vi "Main Board Game.vi"(8 "error in (no error)":errorcluster, 11 "Module_Refs":T1={"ModuleName"=enum."Controller", "Queue"=refnum, "user event"=refnum, "VI Refnum"=refnum, "ShowFP"=FALSE, "StatesTracking Enabled"=FALSE}) -> (0 "error out":errorcluster)   [LabVIEW 2021, in "Board Game.lvlib"]
doc: "Main Module Template of the architecture. Use this as a template to integrate new independent processes into your application."
uses:
  Board Game.lvlib
  Typedefs/Module References.ctl
  Typedefs/Enum_Module_Name.ctl
  Typedefs/Message.ctl
  Typedefs/State Machine Data.ctl
  Typedefs/Config.ctl
  Application/Game.lvclass
  Configuration/Typedefs/App Cfg DVR.ctl
  Typedefs/Application Configuration.ctl
  Module Template/Typedefs/Config.ctl
  Modules/Sound Manager/Typedefs/Config.ctl
  Core UI Configuraton Extractor API.vi
  Configuration/Configuration.lvlib
  Architecture.lvlib
  Module Template/Module Template.lvlib
  Modules/Sound Manager/Sound Manager.lvlib
panel:
  in  "Stop App":bool
  out "Message":string
  in  "Stop Module":bool
  # "#Architecture\n\nPlace inside this box all visible data."
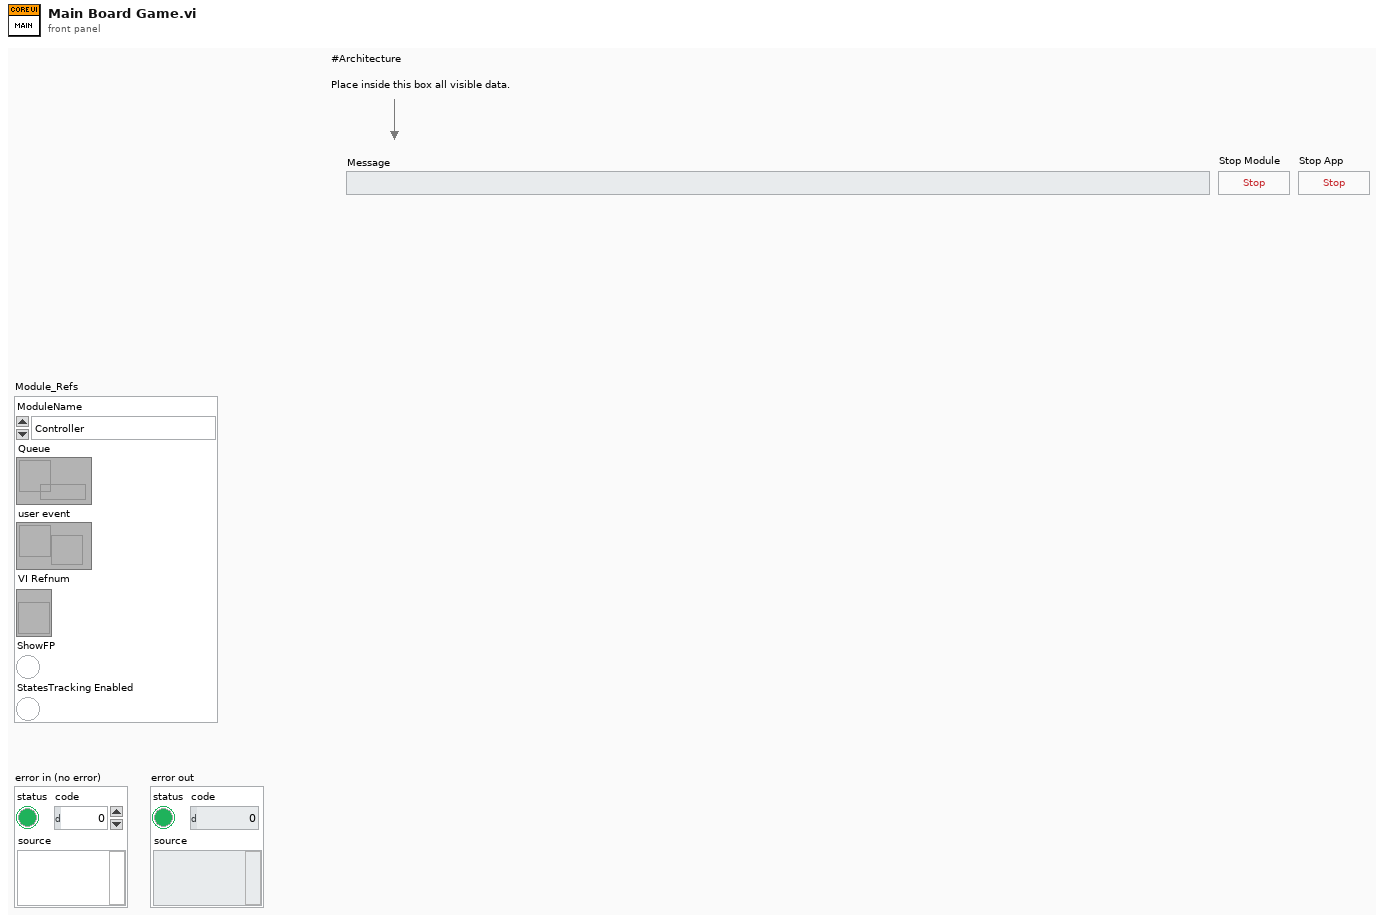
[diagram p1: front panel]
types:
  T1 = typedef "Architecture.lvlib/Module References.ctl" = cluster{"ModuleName":T2, "Queue":refnum<queue>, "user event":refnum<user-event>, "VI Refnum":refnum<vi>, "ShowFP":bool, "StatesTracking Enabled":bool}
  T2 = typedef "Configuration.lvlib/Enum_Module_Name.ctl" = enum16{"Configuration", "Error_Handler", "Log", "Database", "Controller", "UI Module", "Sound Manager"}
  T3 = typedef "Board Game.lvlib/State Machine Data.ctl" = cluster{"Module_Refs":T1, "Response Data":variant, "Core UI Config":T4, "Game":refnum<class "Game.lvclass">}
  T4 = typedef "Board Game.lvlib/Config.ctl" = cluster{"Module Enabled":bool}
  T5 = enum32{"Invalid", "Standard", "Closed", "Hidden", "Minimized", "Maximized"}
  T6 = typedef "Error_Manager.lvlib/LogRotate.lvclass/LogData.ctl" = cluster{"error in":errorcluster, "replacements":string[], "Time Stamp":timestamp}
  T7 = typedef "Configuration.lvlib/App Cfg DVR.ctl" = refnum<data-value>
  T8 = typedef "Module Template.lvlib/Config.ctl" = cluster{"Module Enabled":bool}
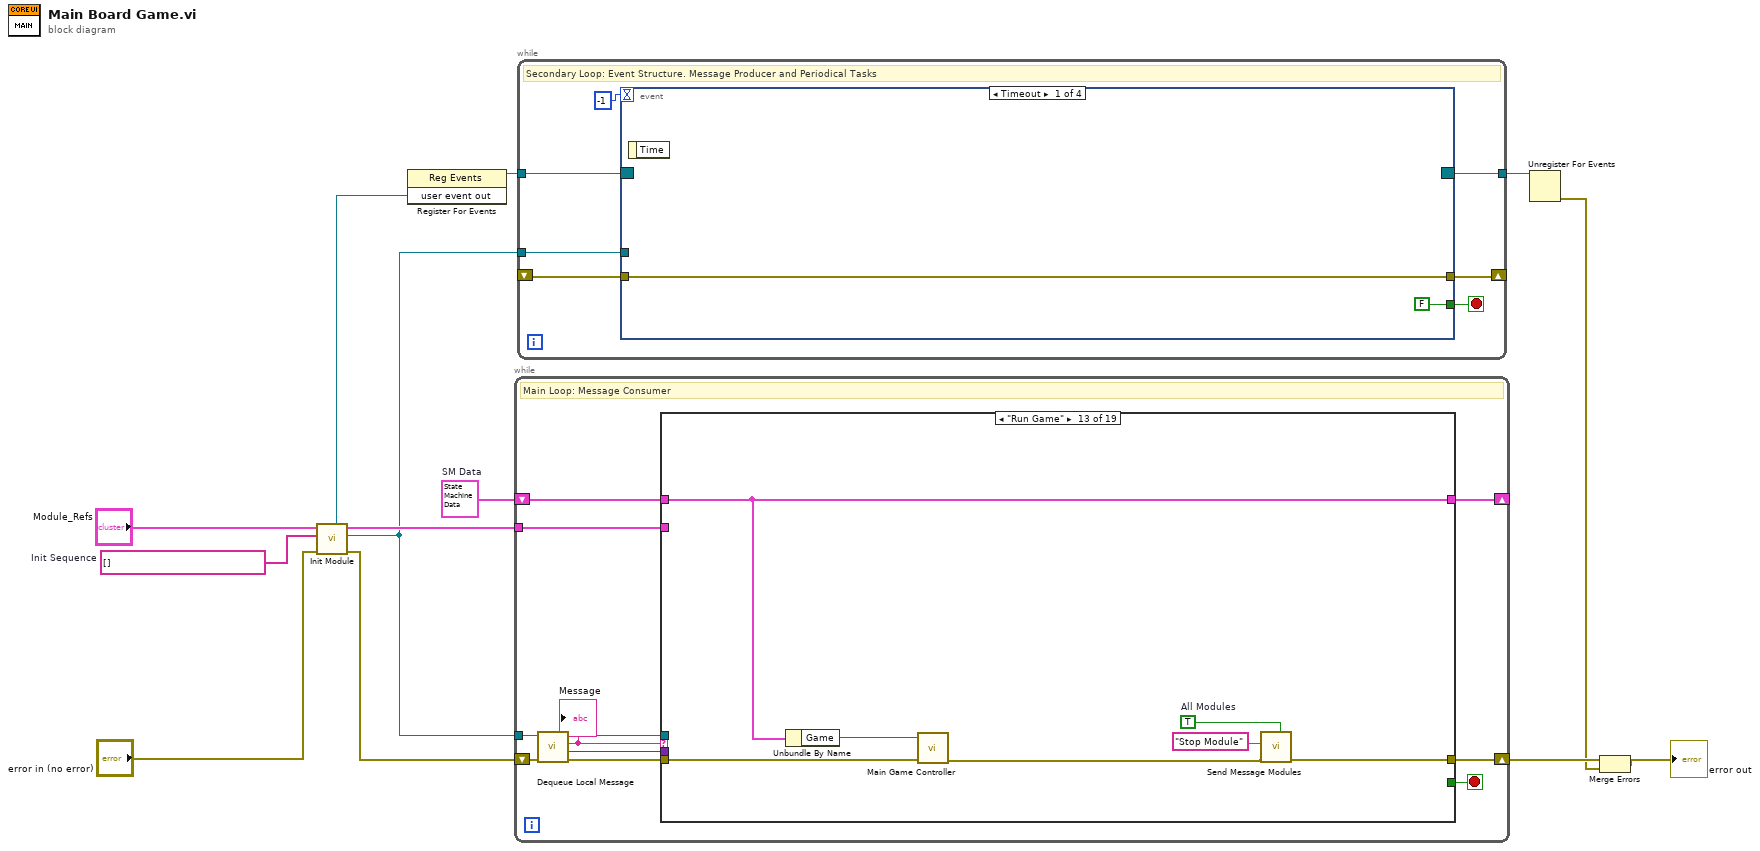
[diagram p0: block diagram]
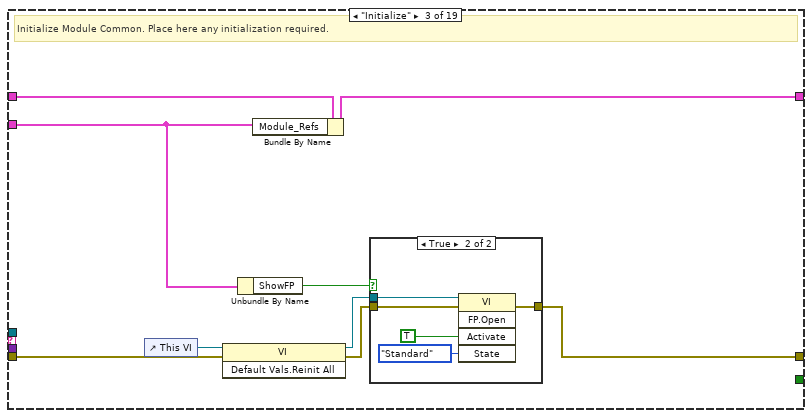
[diagram p4: hidden frame]
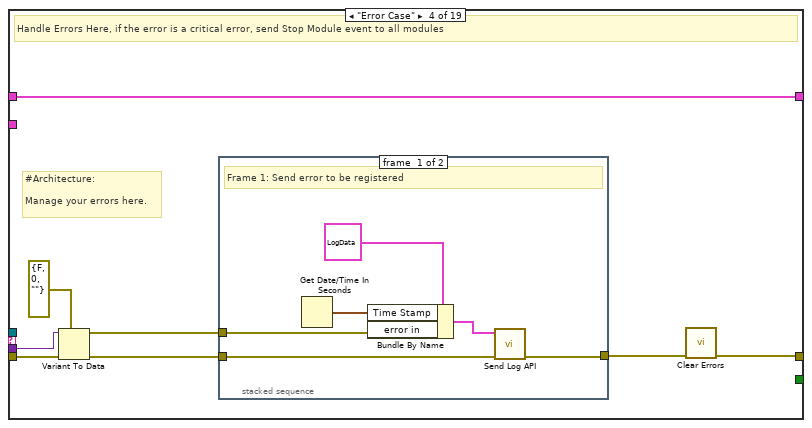
[diagram p6: hidden frame]
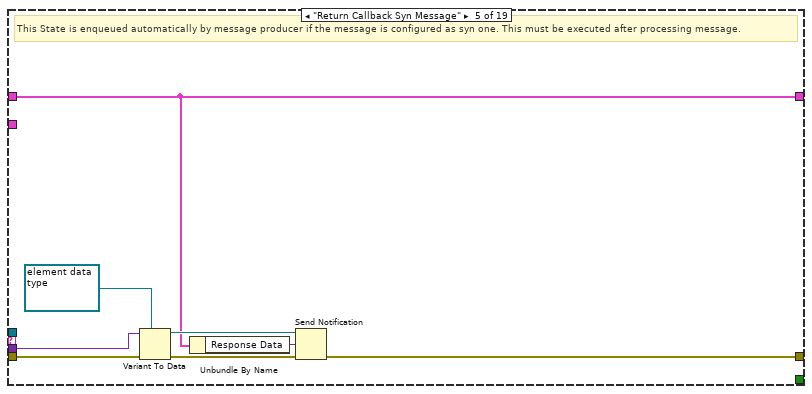
[diagram p9: hidden frame]
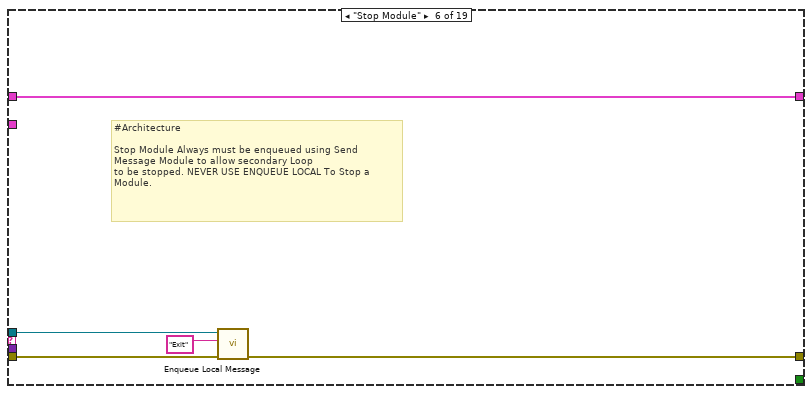
[diagram p10: hidden frame]
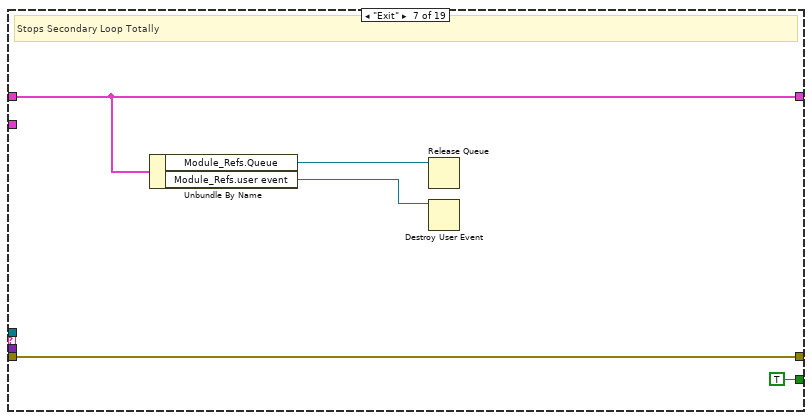
[diagram p11: hidden frame]
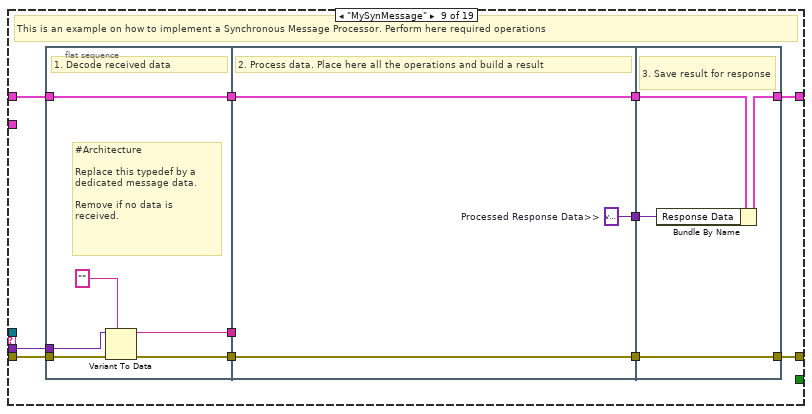
[diagram p13: hidden frame]
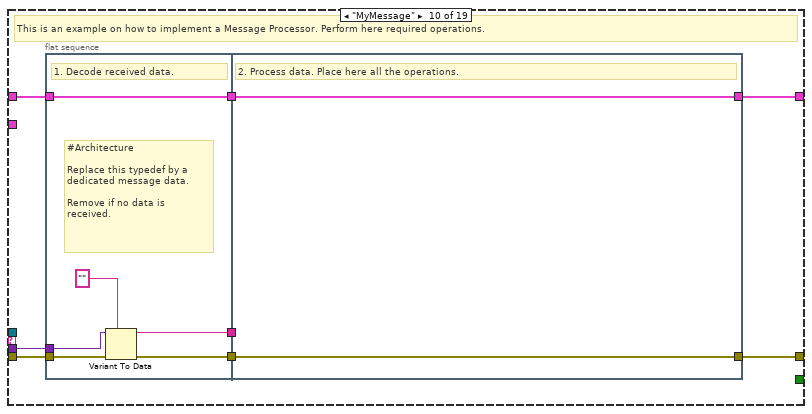
[diagram p14: hidden frame]
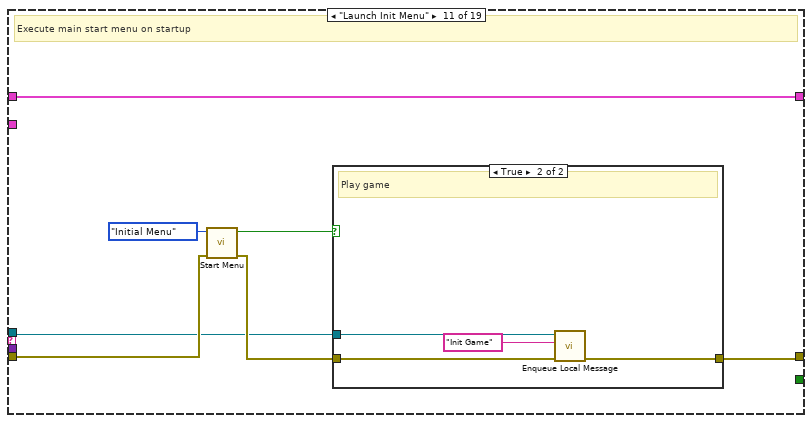
[diagram p15: hidden frame]
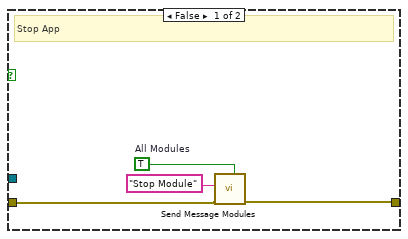
[diagram p16: hidden frame]
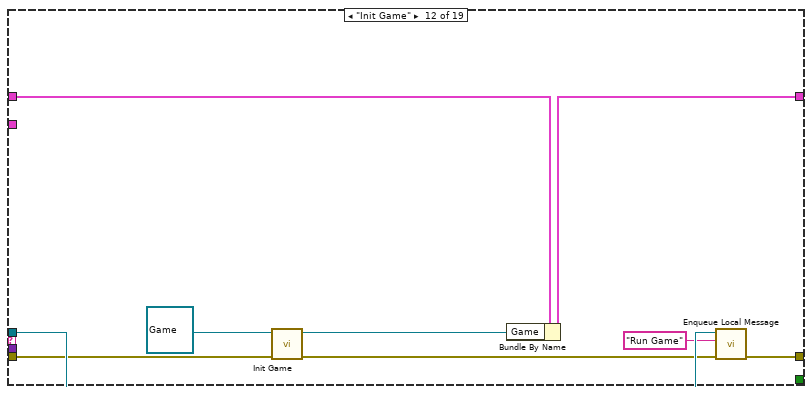
[diagram p17: hidden frame]
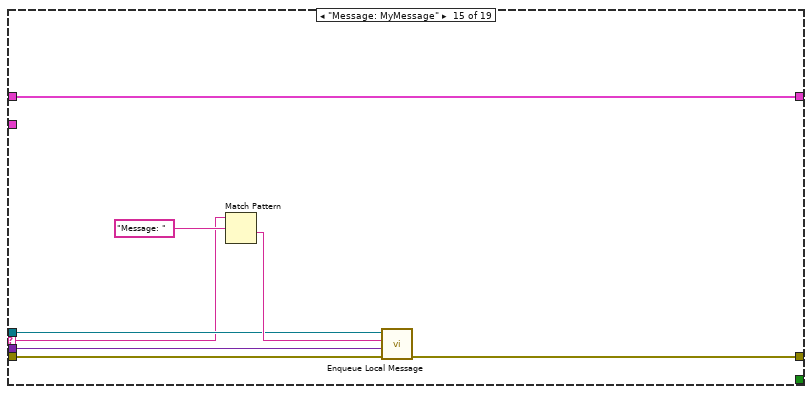
[diagram p19: hidden frame]
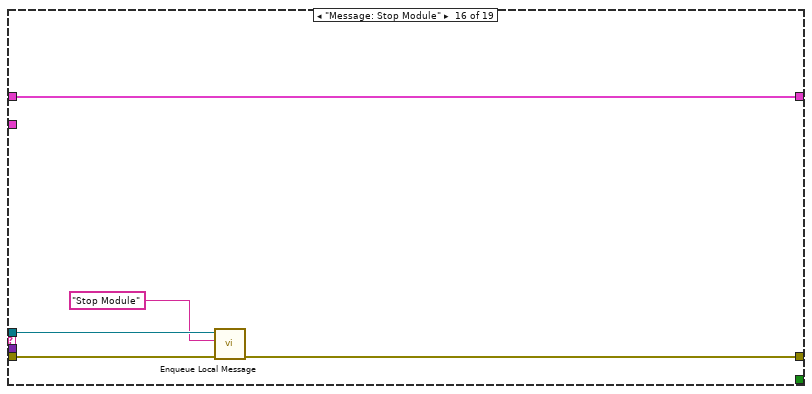
[diagram p20: hidden frame]
diagram:
  w10 = string[] []  # Init Sequence
  w13 = T3 {"Module_Refs"={"ModuleName"=enum."Configuration", "Queue"=refnum, "user event"=refnum, "VI Refnum"=refnum, "ShowFP"=FALSE, "StatesTracking Enabled"=FALSE}, "Response Data"=variant, "Core UI Config"={"Module Enabled"=FALSE}, "Game"=refnum}  # SM Data
  n1 = call "Init Module.vi"("error in (no error)"="error in (no error)", "Init Sequence"=w10, "Module Refs"="Module_Refs") -> ("error out"=w12:errorcluster, "queue out"=w1:refnum<queue>, "Module Refs Out"=w3:T1, "user event out"=w2:refnum<user-event>)  [unwired: 5 in]
  n2 = register-events(w2) -> (reference out=w9:refnum<event-registration>)  [unwired: 2 in, 1 out]
  n3 = while {
    shift-right: [w23] -> _
    shift-left: w13 -> [w24]
    shift-right: [w22] -> w7
    shift-left: w12 -> [w20]
    tunnel: w1 -> [w21]
    tunnel: w3 -> [w14]
    stop <- w15 stop-if-true
    # "Main Loop: Message Consumer"
    n4 = call "Dequeue Local Message.vi"("error in"=w20, "Msg queue in"=w21) -> ("error out"=w19:errorcluster, "Data"=w16:variant, "Message"=w17:string, "queue out"=w18:refnum<queue>)  [unwired: 6 in]
    "Message" <- w17
    n5 = case shown="\"Run Game\"" w17 {
      selector: w17 -> [_ _ _ _ _ _ _ _ _ _ _ _ _ _ w155 _ _ _ w187]
      tunnel: w24 -> [w26 w28 w37 w51 w63 w74 w77 w81 w92 w113 w128 w145 w152 w154 w162 w167 w176 w178 w192]
      tunnel: [w26 w28 w35 w51 w63 w74 w77 w81 w91 w106 w128 w144 w152 w154 w162 w167 w170 w178 w192] -> w23
      tunnel: w19 -> [w25 w27 w36 w50 w69 w73 w79 w80 w85 w109 w127 w138 w147 w153 w159 w166 w175 w177 w191]
      tunnel: [w25 w27 w31 w44 w68 w72 w79 w80 w90 w112 w123 w143 w146 w153 w156 w165 w171 w177 w181] -> w22
      tunnel: w18 -> [_ _ _ _ _ w71 _ _ _ _ w122 w142 _ _ w157 w164 _ _ w188]
      tunnel: w16 -> [_ _ _ w49 w66 _ _ _ w84 w108 _ _ _ _ w158 _ w174 _ w189]
      tunnel: [_ _ _ _ _ _ TRUE _ _ _ _ _ _ _ _ _ _ _ _] -> w15
      tunnel: w14 -> [_ _ w34 _ _ _ _ _ _ _ _ _ _ _ _ _ _ _ _]
      frame "--------State Machine Arquitechture Operations--------" {
      }
      frame "Idle", Default {
        # "Use this state to make iterations if required."
      }
      frame "Initialize" {
        # "Initialize Module Common. Place here any initialization required."
        n6 = control-ref of="This VI"() -> (w29:refnum<vi>)
        n7 = invoke class="VI" method="Default Vals.Reinit All"(reference=w29, error in=w36) -> (reference out=w32:refnum<vi>, error out=w33:errorcluster)  [unwired: 1 in, 1 out]
        n8 = Unbundle By Name(w34) -> ("ShowFP"=w30:bool)
        n9 = Bundle By Name(cluster=w37, "Module_Refs"=w34) -> (w35:T3)
        n10 = case shown="True" w30 {
          tunnel: w33 -> [w38 w43]
          tunnel: [w38 w42] -> w31
          tunnel: w32 -> [_ w41]
          frame False {
          }
          frame True {
            n11 = invoke class="VI" method="FP.Open"(reference=w41, error in=w43, "Activate"=TRUE ("Activate?"), "State"=T5."Standard") -> (error out=w42:errorcluster)  [unwired: 1 in, 4 out]
          }
        }
      }
      frame "Error Case" {
        # "#Architecture: \n\nManage your errors here."
        # "Handle Errors Here, if the error is a critical error, send Stop Module event to all modules"
        n12 = Variant To Data(error in=w50, type=errorcluster {"status"=FALSE, "code"=0, "source"=""} ("error constant"), Variant=w49) -> (data=w45:errorcluster, error out=w47:errorcluster)
        n13 = stacked-sequence {
          tunnel: w47 -> [w57 w59]
          tunnel: [w56 _] -> w46
          tunnel: w45 -> [w54 w58]
          frame #0 {
            # "Frame 1: Send error to be registered"
            n14 = Get Date/Time In Seconds() -> (seconds since 1Jan1904=w53:timestamp)
            n15 = Bundle By Name(cluster=T6 {"error in"={"status"=FALSE, "code"=0, "source"=""}, "replacements"=[], "Time Stamp"=timestamp(0 s since 1904-01-01)} ("Data"), "Time Stamp"=w53, "error in"=w54) -> (w52:T6)
            n16 = call "Send Log API.vi"("error in (no error)"=w57, "Data"=w52) -> ("error out"=w56:errorcluster)  [unwired: 9 in]
          }
          frame #1 {
            # "Frame 2: Manage your errors here"
            n17 = case shown="No Error" w58 {
              tunnel: [w60 w61] -> _
              tunnel: w59 -> [w60 w61]
              frame No Error {
              }
              frame Error {
                # "#Architecture \n\nPlace here critical errors to be managed \nin the desired way."
              }
            }
          }
        }
        n18 = call <vilib>:"Clear Errors.vi"("error in (no error)"=w46) -> ("error out"=w44:errorcluster)  [unwired: 5 in, 1 out]
      }
      frame "Return Callback Syn Message" {
        # "This State is enqueued automatically by message producer if the message is configured as syn one. This must be executed after processing message."
        n19 = Variant To Data(error in=w69, type=refnum<notifier> refnum ("notifier out"), Variant=w66) -> (data=w64:refnum<notifier>, error out=w67:errorcluster)
        n20 = Unbundle By Name(w63) -> ("Response Data"=w62:variant)
        n21 = Send Notification(notification=w62, notifier=w64, error in (no error)=w67) -> (error out=w68:errorcluster)  [unwired: 1 out]
      }
      frame "Stop Module" {
        # "#Architecture\n\nStop Module Always must be enqueued using Send Message Module to allow secondary Loop\nto be stopped. NEVER USE ENQUEUE LOCAL To Stop a Module."
        n22 = call "Enqueue Local Message.vi"("error in"=w73, "Message"="Exit", "Msg queue in"=w71) -> ("error out"=w72:errorcluster)  [unwired: 7 in, 1 out]
      }
      frame "Exit" {
        # "Stops Secondary Loop Totally"
        n23 = Unbundle By Name(w77) -> ("Module_Refs.Queue"=w76:refnum<queue>, "Module_Refs.user event"=w75:refnum<user-event>)
        n24 = Release Queue(queue=w76) -> ()  [unwired: 2 in, 3 out]
        n25 = Destroy User Event(user event=w75) -> ()  [unwired: 1 in, 1 out]
      }
      frame "--------------State Machine Custom States-------------" {
      }
      frame "MySynMessage" {
        # "This is an example on how to implement a Synchronous Message Processor. Perform here required operations"
        n26 = flat-sequence {
          tunnel: w85 -> [w96]
          tunnel: w92 -> [w98]
          tunnel: [w98] -> w89
          tunnel: [w94] -> w88
          tunnel: w84 -> [w95]
          tunnel: [w93] -> w83
          tunnel: w89 -> [w101]
          tunnel: w88 -> [w100]
          tunnel: [w101] -> w87
          tunnel: [w100] -> w86
          tunnel: w83 -> [_]
          tunnel: [w99] -> w82
          tunnel: [w104] -> w90
          tunnel: [w103] -> w91
          tunnel: w87 -> [w105]
          tunnel: w86 -> [w104]
          tunnel: w82 -> [w102]
          frame #0 {
            # "#Architecture\n\nReplace this typedef by a dedicated message data.\n\nRemove if no data is received."
            # "1. Decode received data"
            n27 = Variant To Data(error in=w96, type="", Variant=w95) -> (data=w93:string, error out=w94:errorcluster)
          }
          frame #1 {
            w99 = variant  # Processed Response Data>>
            # "2. Process data. Place here all the operations and build a result"
          }
          frame #2 {
            # "3. Save result for response"
            n28 = Bundle By Name(cluster=w105, "Response Data"=w102) -> (w103:T3)
          }
        }
      }
      frame "MyMessage" {
        # "This is an example on how to implement a Message Processor. Perform here required operations."
        n29 = flat-sequence {
          tunnel: w109 -> [w117]
          tunnel: w113 -> [w119]
          tunnel: [w119] -> w111
          tunnel: [w115] -> w110
          tunnel: w108 -> [w116]
          tunnel: [w114] -> w107
          tunnel: w111 -> [w120]
          tunnel: w110 -> [w121]
          tunnel: w107 -> [_]
          tunnel: [w121] -> w112
          tunnel: [w120] -> w106
          frame #0 {
            # "#Architecture\n\nReplace this typedef by a dedicated message data.\n\nRemove if no data is received."
            # "1. Decode received data."
            n30 = Variant To Data(error in=w117, type="", Variant=w116) -> (data=w114:string, error out=w115:errorcluster)
          }
          frame #1 {
            # "2. Process data. Place here all the operations."
          }
        }
      }
      frame "Launch Init Menu" {
        # "Execute main start menu on startup"
        n31 = call "Start Menu.vi"("error in (no error)"=w127, "Enum"=enum16{"Initial Menu", "Final Menu"}."Initial Menu") -> ("error out"=w125:errorcluster, "Start/Stop"=w124:bool)  [unwired: 8 in]
        n32 = case shown="True" w124 {
          tunnel: w125 -> [w130 w136]
          tunnel: [w129 w135] -> w123
          tunnel: w122 -> [_ w134]
          frame False {
            w132 = TRUE  # All Modules
            # "Stop App"
            n33 = call "Send Message Modules.vi"("All Modules"=w132, "Error In"=w130, "Message"="Stop Module") -> ("error in (no error)"=w129:errorcluster)  [unwired: 8 in]
          }
          frame True {
            # "Play game"
            n34 = call "Enqueue Local Message.vi"("error in"=w136, "Message"="Init Game", "Msg queue in"=w134) -> ("error out"=w135:errorcluster)  [unwired: 7 in, 1 out]
          }
        }
      }
      frame "Init Game" {
        n35 = call "Init Game.vi"("error in"=w138, "Game in"=refnum<class "Game.lvclass"> refnum ("input cluster")) -> ("error out"=w137:errorcluster, "Game out"=w139:refnum<class "Game.lvclass">)  [unwired: 8 in]
        n36 = Bundle By Name(cluster=w145, "Game"=w139) -> (w144:T3)
        n37 = call "Enqueue Local Message.vi"("error in"=w137, "Message"="Run Game", "Msg queue in"=w142) -> ("error out"=w143:errorcluster)  [unwired: 7 in, 1 out]
      }
      frame "Run Game" {
        w150 = TRUE  # All Modules
        n38 = Unbundle By Name(w152) -> ("Game"=w151:refnum<class "Game.lvclass">)
        n39 = call "Main Game Controller.vi"("error in (no error)"=w147, "output cluster"=w151) -> ("error out"=w148:errorcluster)  [unwired: 9 in]
        n40 = call "Send Message Modules.vi"("All Modules"=w150, "Error In"=w148, "Message"="Stop Module") -> ("error in (no error)"=w146:errorcluster)  [unwired: 8 in]
      }
      frame "--------------Dynamic Events Messages----------------" {
      }
      frame "Message: MyMessage" {
        n41 = Match Pattern(string=w155, regular expression="Message: ") -> (after substring=w160:string)  [unwired: 1 in, 3 out]
        n42 = call "Enqueue Local Message.vi"("error in"=w159, "Data"=w158, "Message"=w160, "Msg queue in"=w157) -> ("error out"=w156:errorcluster)  [unwired: 6 in, 1 out]
      }
      frame "Message: Stop Module" {
        n43 = call "Enqueue Local Message.vi"("error in"=w166, "Message"="Stop Module", "Msg queue in"=w164) -> ("error out"=w165:errorcluster)  [unwired: 7 in, 1 out]
      }
      frame "Message: Load Config" {
        # "Get dedicated data for this module from \ngeneral DVR configuration and save it into \nSM Data to use it on runtime."
        # "Message used to receive configuration from a configuration module. Decode dedicated typedef and save it into SM Data"
        n44 = Variant To Data(error in=w175, type=T7 refnum ("App Cfg DVR"), Variant=w174) -> (data=w173:T7, error out=w172:errorcluster)
        n45 = call-poly "POLY Read Configuration API.vi"("error constant"=w172, "App Cfg DVR"=w173) -> ("error out"=w171:errorcluster, "Module Template Config"=w169:T8)  [unwired: 8 in]
        n46 = Bundle By Name(cluster=w176, "Core UI Config"=w169) -> (w170:T3)
      }
      frame "------------Synchronous Event Messages--------------" {
      }
      frame "SynMessage: Launch Init Menu", "SynMessage: MySynMessage" {
        # "Use this case as a handler for Synchronous messages. This state queues a message for the desired"
        n47 = call "Extract Synchronous Data.vi"("error in 2"=w191, "Variant"=w189) -> ("error in"=w190:errorcluster, "Data Out"=w184:variant, "notifier out"=w179:refnum<notifier>)  [unwired: 7 in]
        n48 = Match Pattern(string=w187, regular expression="SynMessage: ") -> (after substring=w185:string)  [unwired: 1 in, 3 out]
        n49 = call "Enqueue Local Message.vi"("error in"=w190, "Data"=w184, "Message"=w185, "Msg queue in"=w188) -> ("error out"=w183:errorcluster, "queue out"=w182:refnum<queue>)  [unwired: 6 in]
        n50 = call "Enqueue Local Message.vi"("error in"=w183, "Data"=w179, "Message"="Return Callback Syn Message", "Msg queue in"=w182) -> ("error out"=w181:errorcluster)  [unwired: 6 in, 1 out]
      }
    }
  }
  n51 = while {
    tunnel: w9 -> [w199]
    tunnel: w1 -> [w196]
    tunnel: [w195] -> w8
    shift-right: [w193] -> _
    shift-left: _ -> [w194]
    stop <- w197 stop-if-true
    # "Secondary Loop: Event Structure. Message Producer and Periodical Tasks"
    n52 = event shown="[0] Timeout" {
      selector: w199 -> [_ _ _ _]
      dyn-events: [_ _ _ _] -> w195
      timeout: -1 -> [_ _ _ _]
      tunnel: [FALSE w208 TRUE _] -> w197
      tunnel: w196 -> [_ w213 w215 _]
      tunnel: w194 -> [w200 w212 w218 w220]
      tunnel: [w200 w211 w216 w219] -> w193
      event Timeout {
        n53 = event-data() -> ()  [unwired: 1 in, 1 out]
      }
      event User Event {
        # "Send message to local queue. \n(Message Consumer)"
        # "Processes an external event and enqueues a message to the local queue. It can be synchronous (with response) or NOT."
        n54 = event-data() -> ("syn"=w205:bool, "Message"=w207:string, "Data"=w210:variant)  [unwired: 1 in]
        n55 = Select(t="SynMessage: " ("string"), s=w205, f="Message: " ("string")) -> (s? t:f=w202:string)
        n56 = Concatenate Strings(w202, w207) -> (w209:string)
        n57 = call "Enqueue Local Message.vi"("error in"=w212, "Data"=w210, "Message"=w209, "Msg queue in"=w213) -> ("error out"=w211:errorcluster)  [unwired: 6 in, 1 out]
        n58 = Equal?(x=w207, y="Stop Module") -> (x = y?=w208:bool)
      }
      event "Stop Module": Value Change {
        n59 = event-data() -> ()  [unwired: 1 in, 1 out]
        n60 = call "Enqueue Local Message.vi"("error in"=w218, "Message"="Stop Module", "Msg queue in"=w215) -> ("error out"=w216:errorcluster)  [unwired: 7 in, 1 out]
      }
      event "Stop App": Value Change {
        w222 = TRUE  # All Modules
        # "Send Stop To All Modules"
        n61 = event-data() -> ()  [unwired: 1 in, 1 out]
        n62 = call "Send Message Modules.vi"("All Modules"=w222, "Error In"=w220, "Message"="Stop Module") -> ("error in (no error)"=w219:errorcluster)  [unwired: 8 in]
      }
    }
  }
  n63 = Unregister For Events(event registration refnum=w8) -> (error out=w6:errorcluster)  [unwired: 1 in]
  n64 = Merge Errors(w7, w6) -> (→"error out":errorcluster)
